vi "Populate and conf ethernet bus.vi"(8 "Error In":errorcluster, 9 "Empty buffer":bool) -> (0 "Error Out":errorcluster, 3 "Devices":refnum<visa-resource-name>[](array[refnum]))   [LabVIEW 2015]
uses:
  <vilib>/Instr/_visa.llb/VISA Find Search Mode.ctl
  <vilib>/Utility/error.llb/Error Cluster From Error Code.vi
  <vilib>/ErrorRing/Error Ring.xnode
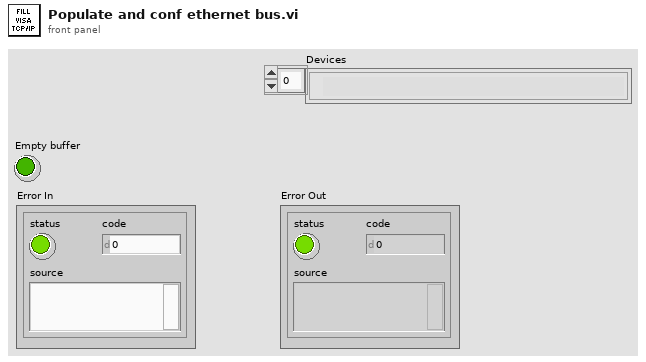
[diagram p1: front panel]
types:
  T1 = typedef "VISA Find Search Mode.ctl" = u32
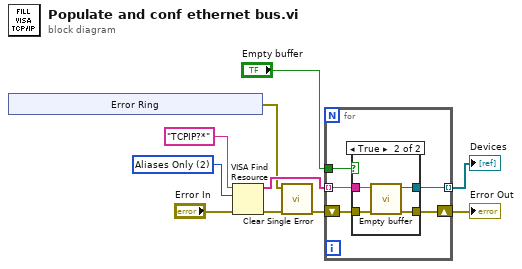
[diagram p0: block diagram]
diagram:
  w10 = T1 2 items=["Canonical Names Only"=0, "Aliases Only"=2, "Include Matching Aliases"=3, "Include All Aliases"=4] ("Search Mode")
  n1 = xnode "Error Ring"() -> ("error out"=w1:errorcluster)
  n2 = VISA Find Resource(8:"Error In", 10:w10, 11:"TCPIP?*" ("expression (\"?*\")")) -> (0:w7:errorcluster, 3:w8:string[])  [unwired: 1 out]
  n3 = call "Clear Single Error.vi"("Error In"=w7, "Error to clear"=w1) -> ("Error Out"=w2:errorcluster)  [unwired: 8 in, 1 out]
  n4 = for {
    tunnel: w8 -> [w15] mode=indexing
    tunnel: [w11] -> w6 mode=indexing
    shift-right: [w12] -> w4
    shift-left: w2 -> [w14]
    tunnel: "Empty buffer" -> [w13]
    n5 = case shown="True" w13 {
      tunnel: w14 -> [w16 w21]
      tunnel: [w16 w20] -> w12
      tunnel: w15 -> [w17 w19]
      tunnel: [w17 w18] -> w11
      frame False {
      }
      frame True {
        n6 = call "Empty buffer.vi"("Error In"=w21, "VISA resource name"=w19) -> ("Error Out"=w20:errorcluster, "VISA resource name out"=w18:refnum<visa-resource-name>)  [unwired: 7 in, 1 out]
      }
    }
  }
  "Devices" <- w6
  "Error Out" <- w4
